vi "test_AK TCP_AK TCP Write.vi"(8 "error in (no error)":errorcluster, 11 "TestCase in":refnum<class "Ethernet Protocol Tests.lvclass">) -> (0 "error out":errorcluster, 3 "TestCase out":refnum<class "Ethernet Protocol Tests.lvclass">)   [LabVIEW 2019, in "Ethernet Protocol Tests.lvclass"]
uses:
  Ethernet Protocol Tests.lvclass
  Listener/Listener.lvclass
  Listener/ListenerClassControls/Operation.ctl
  AK TCP/AK TCP.lvclass
  D:/GitRepository/niveristand-instrument-addon-classes/Source/Protocols/TCP/TCP.lvclass
  D:/GitRepository/niveristand-instrument-addon-classes/Source/Protocols/Protocol Parent/Protocol Parent.lvclass
  TCP/TCP.lvclass/TCP.ctl
  Listener/ListenerClassMethods/Constants.vi
  <vilib>/addons/_JKI Toolkits/VI Tester/TestCase.llb/TestCase.lvclass
  TCP/TCP.lvclass
  C:/Program Files (x86)/National Instruments/LabVIEW 2019/vi.lib/addons/_JKI Toolkits/VI Tester/TestCase.llb/TestCase.lvclass
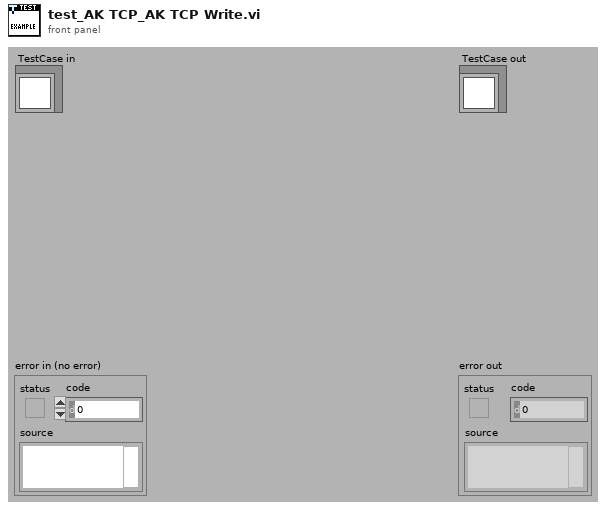
[diagram p1: front panel]
types:
  T1 = typedef "Listener.lvclass/Operation.ctl" = enum16{"Read", "Write"}
  T2 = typedef "Listener.lvclass/AK TCP Data Structure.ctl" = cluster{"TCP|IP connection ID":refnum<k5>, "IP Address":string, "Port":u16, "Data":string, "Current Command Code":string}
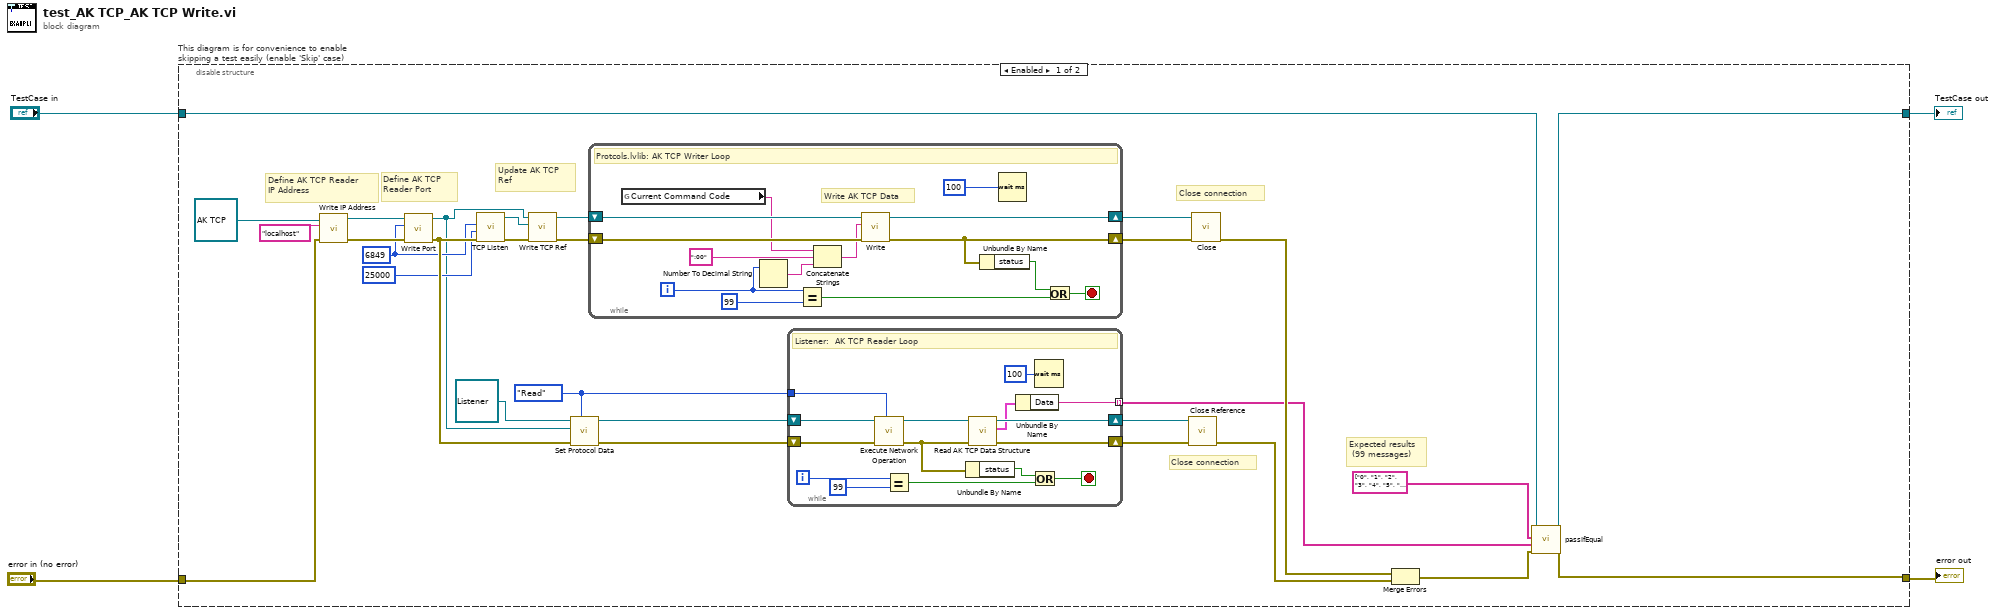
[diagram p0: block diagram]
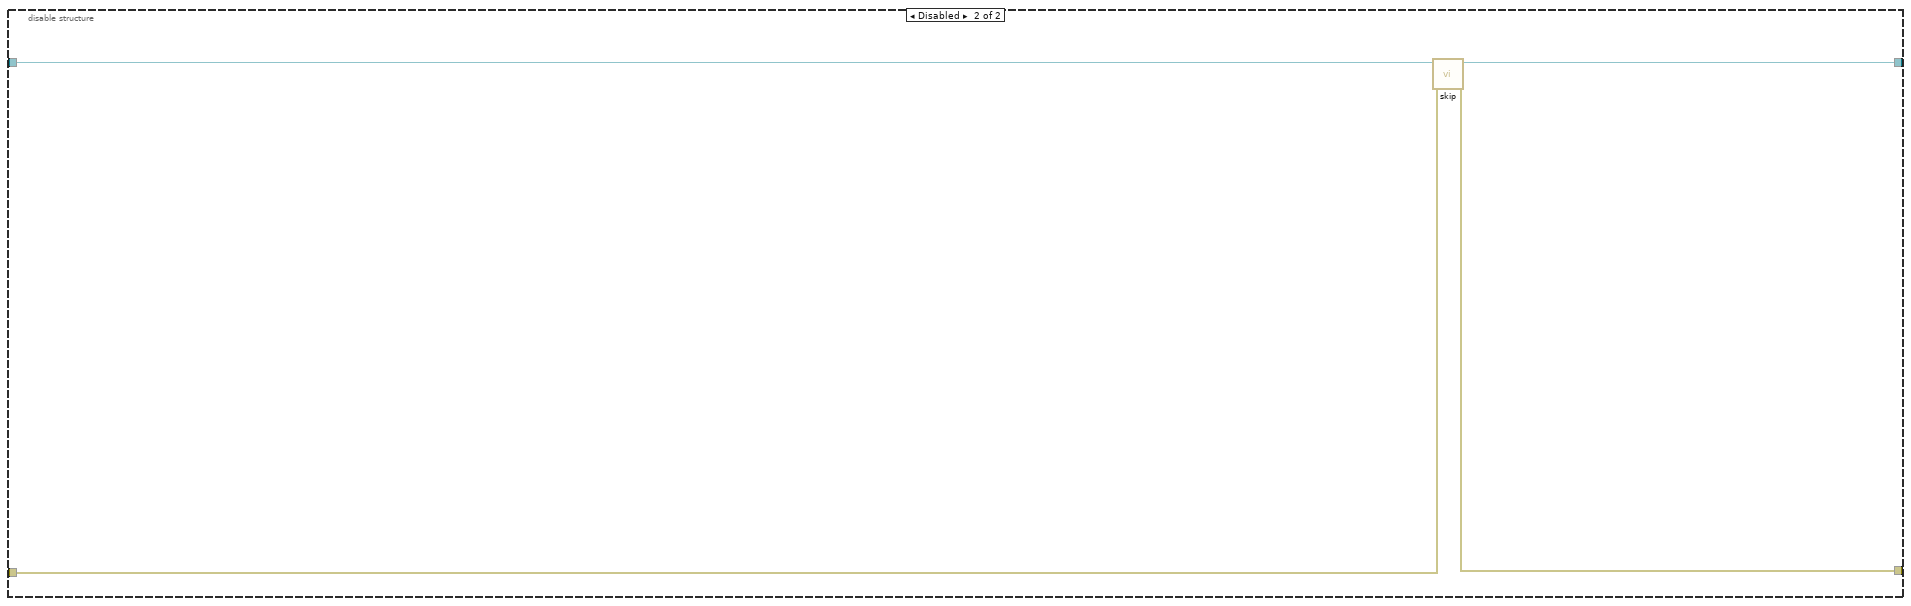
[diagram p2: hidden frame]
diagram:
  n1 = disable-structure "This diagram is for convenience to enable skipping a test easily (enable 'Skip' case)" shown="Enabled" {
    disable-tunnel: "TestCase in" -> [w33 w66]
    disable-tunnel: [w32 w64] -> w1
    disable-tunnel: [w31 w65] -> w3
    disable-tunnel: "error in (no error)" -> [w27 w63]
    frame Enabled {
      w14 = Operation."Read" ("Operation")
      w21 = u16 6849 ("Port")
      # "Close connection"
      # "Close connection"
      # "Update AK TCP \nRef"
      # "Expected results\n (99 messages)"
      # "Define AK TCP \nReader Port"
      # "Define AK TCP Reader \nIP Address"
      n2 = call "Write IP Address.vi"("error in (no error)"=w27, "IP Address"="localhost", "Ethernet in"=refnum<class "AK TCP.lvclass"> refnum ("Protocols.lvlib:AK TCP.lvclass")) -> ("error out"=w28:errorcluster, "Ethernet out"=w29:refnum<class "AK TCP.lvclass">)  [unwired: 7 in]
      n3 = call "Write Port.vi"("error in (no error)"=w28, "Port"=w21, "Ethernet in"=w29) -> ("error out"=w22:errorcluster, "Ethernet out"=w16:refnum<class "AK TCP.lvclass">)  [unwired: 7 in]
      n4 = call <vilib>:"TCP Listen.vi"("error in (no error)"=w22, "timeout ms (wait forever: -1)"=25000, "port"=w21) -> ("error out"=w19:errorcluster, "connection ID"=w15:refnum<k5>)  [unwired: 4 in, 3 out]
      n5 = call "Write TCP Ref.vi"("error in (no error)"=w19, "TCP Ref"=w15, "Ethernet in"=w16) -> ("error out"=w18:errorcluster, "Ethernet out"=w17:refnum<class "AK TCP.lvclass">)  [unwired: 7 in]
      n6 = call "Set Protocol Data.vi"("Operation"=w14, "error in (no error)"=w22, "Protocols.lvlib:Protocol Parent.lvclass"=w16, "Listener In.lvclass"=refnum<class "Listener.lvclass"> refnum ("Listener.lvclass")) -> ("error out"=w23:errorcluster, "Listener Out.lvclass"=w24:refnum<class "Listener.lvclass">)  [unwired: 6 in]
      n7 = while {
        shift-right: [w56] -> w10
        shift-left: w18 -> [w54]
        shift-right: [w57] -> w9
        shift-left: w17 -> [w58]
        i -> [w53]
        stop <- w61 stop-if-true
        # "Write AK TCP Data"
        # "Protcols.lvlib: AK TCP Writer Loop"
        n8 = global read "Constants.vi" "Current Command Code"() -> (w52:string)
        n9 = Number To Decimal String(number=w53) -> (decimal integer string=w51:string)  [unwired: 1 in]
        n10 = Equal?(x=w53, y=99 ("x")) -> (x = y?=w62:bool)
        n11 = Concatenate Strings(w52, ":00" ("string"), w51) -> (w49:string)
        n12 = call-dynamic "Write.vi"("error in (no error)"=w54, "String"=w49, "AK TCP in"=w58) -> ("error out"=w56:errorcluster, "AK TCP out"=w57:refnum<class "AK TCP.lvclass">)  [unwired: 7 in]
        n13 = Unbundle By Name(w56) -> ("status"=w55:bool)
        n14 = Wait (ms)(milliseconds to wait=u32 100) -> ()  [unwired: 1 out]
        n15 = Or(x=w55, y=w62) -> (x .or. y?=w61:bool)
      }
      n16 = while {
        shift-right: [w36] -> w12
        shift-left: w23 -> [w48]
        shift-right: [w35] -> w13
        shift-left: w24 -> [w47]
        tunnel: w14 -> [w42]
        tunnel: [w41] -> w7 mode=indexing
        i -> [w40]
        stop <- w45 stop-if-true
        # "Listener:  AK TCP Reader Loop"
        n17 = call "Execute Network Operation.vi"("Operation"=w42, "error in (no error)"=w48, "Listener In.lvclass"=w47) -> ("error out"=w38:errorcluster, "Listener Out.lvclass"=w37:refnum<class "Listener.lvclass">)  [unwired: 7 in]
        n18 = Equal?(x=w40, y=99 ("x")) -> (x = y?=w44:bool)
        n19 = Unbundle By Name(w38) -> ("status"=w46:bool)
        n20 = call-dynamic "Read AK TCP Data Structure.vi"("error in (no error)"=w38, "Listener in"=w37) -> ("error out"=w36:errorcluster, "TCP|IP Data Structure"=w34:T2, "Listener out"=w35:refnum<class "Listener.lvclass">)  [unwired: 7 in]
        n21 = Unbundle By Name(w34) -> ("Data"=w41:string)
        n22 = Or(x=w46, y=w44) -> (x .or. y?=w45:bool)
        n23 = Wait (ms)(milliseconds to wait=u32 100) -> ()  [unwired: 1 out]
      }
      n24 = call "Close Reference.vi"("error in (no error)"=w12, "Listener In.lvclass"=w13) -> ("error out"=w11:errorcluster)  [unwired: 9 in]
      n25 = call-dynamic "Close.vi"("error in (no error)"=w10, "Ethernet in"=w9) -> ("error out"=w8:errorcluster)  [unwired: 8 in, 1 out]
      n26 = Merge Errors(w8, w11) -> (w26:errorcluster)
      n27 = call-dynamic "passIfEqual.vi"("error in (no error)"=w26, "y"=w7, "x"=string[] ["0", "1", "2", "3", "4", "5", "6", "7", "8", "9", "10", "11", "12", "13", "14", "15", "16", "17", "18", "19", "20", "21", "22", "23", "24", "25", "26", "27", "28", "29", "30", "31", "32", "33", "34", "35", "36", "37", "38", "39", "40", "41", "42", "43", "44", "45", "46", "47", "48", "49", "50", "51", "52", "53", "54", "55", "56", "57", "58", "59", "60", "61", "62", "63", "64", "65", "66", "67", "68", "69", "70", "71", "72", "73", "74", "75", "76", "77", "78", "79", "80", "81", "82", "83", "84", "85", "86", "87", "88", "89", "90", "91", "92", "93", "94", "95", "96", "97", "98", "99"] ("Array"), "TestCase in"=w33) -> ("error out"=w31:errorcluster, "TestCase out"=w32:refnum<class "Ethernet Protocol Tests.lvclass">)  [unwired: 6 in]
    }
    frame Disabled {
      # "skip test result while test is under development"
      n28 = call <vilib>:"skip.vi"("error in (no error)"=w63, "TestCase in"=w66) -> ("error out"=w65:errorcluster, "TestCase out"=w64:refnum<class "Ethernet Protocol Tests.lvclass">)  [unwired: 8 in]
    }
  }
  "error out" <- w3
  "TestCase out" <- w1
